vi "tarcfg serialize test.vi"() -> ()   [LabVIEW 2014, in "configuration tests.lvlib"]
uses:
  configuration tests.lvlib
  Framework Configuration Classes/target configuration/PL_Target Configuration.lvclass
  <vilib>/NI/Tag Bus Module Framework/root configuration/Target Types.ctl
  <vilib>/NI/Configuration Framework/serializable configuration/NISE_CEF_serializable configuration.lvclass/NISE_CEF_serializable configuration.ctl
  Framework Configuration Classes/target configuration/PL_Target Configuration.lvclass/PL_Target Configuration.ctl
  <vilib>/NI/Configuration Framework/serializable configuration/Read UID.vi
  Framework Configuration Classes/target configuration/Write hostname.vi
  Framework Configuration Classes/target configuration/Write name.vi
  Framework Configuration Classes/target configuration/Write OS.vi
  Framework Configuration Classes/target configuration/Write Config Path.vi
  Framework Configuration Classes/target configuration/Write load bitfile.vi
  Framework Configuration Classes/target configuration/Write RIO FPGA.vi
  Framework Configuration Classes/target configuration/Write bitfile path.vi
  Framework Configuration Classes/target configuration/Read hostname.vi
  Framework Configuration Classes/target configuration/Read name.vi
  Framework Configuration Classes/target configuration/Read OS.vi
  Framework Configuration Classes/target configuration/Read Config Path.vi
  Framework Configuration Classes/target configuration/Read load bitfile.vi
  Framework Configuration Classes/target configuration/Read RIO FPGA.vi
  Framework Configuration Classes/target configuration/Read bitfile path.vi
  <vilib>/Utility/LVClass/Get LV Class Name.vi
  <vilib>/NI/Configuration Framework/error generator/NISE_error generator.vi
  <vilib>/NI/Configuration Framework/serializable configuration/set alias.vi
  <vilib>/NI/Configuration Framework/serializable configuration/get alias.vi
  <vilib>/NI/Configuration Framework/serializable configuration/NISE_CEF_serializable configuration.lvclass
  <vilib>/NI/Tag Bus Module Framework/root configuration/TBM configuration.lvclass
panel:
  out "loadbit ok":bool
  out "rio ok":bool
  out "bitfile ok":bool
  out "pathok":bool
  out "OSok":bool
  out "nameok":bool
  out "hostok":bool
  out "idok":bool
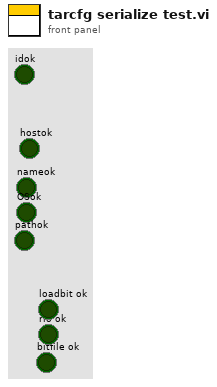
[diagram p1: front panel]
types:
  T1 = typedef "TBM configuration.lvclass/Target Types.ctl" = enum16{"Windows", "Mac", "Linux", "Linux RT ARM", "VxWorks", "Pharlap", "Other", "Linux RT x64"}
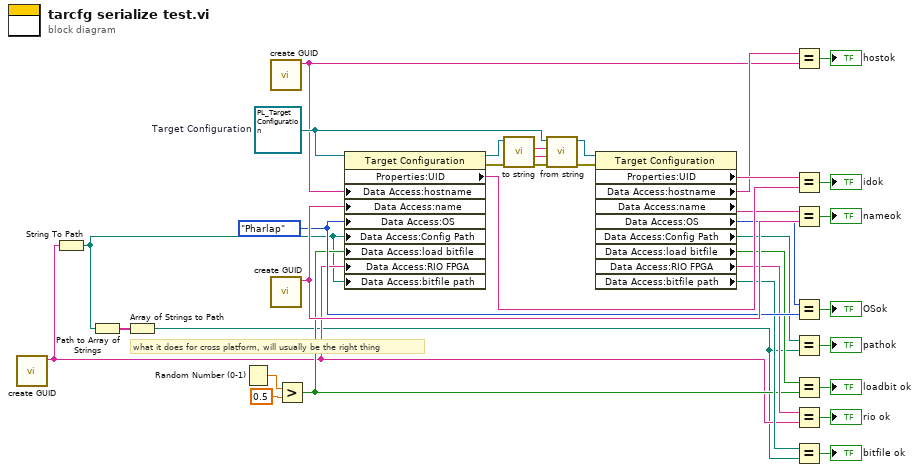
[diagram p0: block diagram]
diagram:
  w15 = Target_Types."Pharlap" ("OS")
  w22 = refnum<class "PL_Target Configuration.lvclass"> refnum  # Target Configuration
  # "what it does for cross platform, will usually be the right thing"
  n1 = call <vilib>:"create GUID.vi"() -> ("uuid"=w3:string)  [unwired: 10 in, 1 out]
  n2 = String To Path(string=w3) -> (path=w2:path)
  n3 = Path to Array of Strings(0:w2) -> (2:w13:string[])  [unwired: 1 out]
  n4 = Array of Strings to Path(0:w13) -> (2:w1:path)  [unwired: 1 in]
  n5 = Random Number (0-1)() -> (number: 0 to 1=w12:dbl)
  n6 = call <vilib>:"create GUID.vi"() -> ("uuid"=w20:string)  [unwired: 10 in, 1 out]
  n7 = call <vilib>:"create GUID.vi"() -> ("uuid"=w25:string)  [unwired: 10 in, 1 out]
  n8 = Greater?(x=w12, y=0.5) -> (0:w4:bool)
  n9 = property class="Target Configuration"(reference=w22, "Data Access:hostname"=w20, "Data Access:name"=w25, "Data Access:OS"=w15, "Data Access:Config Path"=w2, "Data Access:load bitfile"=w4, "Data Access:RIO FPGA"=w3, "Data Access:bitfile path"=w2) -> (reference out=w33:refnum<class "PL_Target Configuration.lvclass">, error out=w24:errorcluster, "Properties:UID"=w29:string)  [unwired: 1 in]
  n10 = call-dynamic "to string.vi"("error in"=w24, "configuration in"=w33) -> ("error out"=w23:errorcluster, "data"=w34:string, "version"=w35:string)  [unwired: 6 in, 1 out]
  n11 = call-dynamic "from string.vi"("error in"=w23, "data"=w34, "version"=w35, "configuration in"=w22) -> ("error out"=w32:errorcluster, "configuration out"=w31:refnum<class "PL_Target Configuration.lvclass">)  [unwired: 6 in]
  n12 = property class="Target Configuration"(reference=w31, error in=w32) -> ("Properties:UID"=w30:string, "Data Access:hostname"=w21:string, "Data Access:name"=w19:string, "Data Access:OS"=w16:T1, "Data Access:Config Path"=w14:path, "Data Access:load bitfile"=w5:bool, "Data Access:RIO FPGA"=w6:string, "Data Access:bitfile path"=w7:path)  [unwired: 2 out]
  n13 = Equal?(x=w21, y=w20) -> (x = y?=→"hostok":bool)
  n14 = Equal?(x=w30, y=w29) -> (x = y?=→"idok":bool)
  n15 = Equal?(x=w19, y=w25) -> (x = y?=→"nameok":bool)
  n16 = Equal?(x=w16, y=w15) -> (x = y?=→"OSok":bool)
  n17 = Equal?(x=w14, y=w1) -> (x = y?=→"pathok":bool)
  n18 = Equal?(x=w5, y=w4) -> (x = y?=→"loadbit ok":bool)
  n19 = Equal?(x=w6, y=w3) -> (x = y?=→"rio ok":bool)
  n20 = Equal?(x=w7, y=w1) -> (x = y?=→"bitfile ok":bool)
